vi "RSZVB Delete All Pulse Train Segments.vi"(8 "error in (no error)":errorcluster {"code" format="%.0x"}, 10 "Channel (1)":i32=1, 11 "VISA session":refnum<visa-resource-name>) -> (0 "error out":errorcluster {"code" format="%.0x"}, 3 "dup VISA session":refnum<visa-resource-name>)   [LabVIEW 2011]
doc: "This VI deletes all pulse train segments..\n\nNote(s):\n\n(1) This VI is available only with option R&S ZVA-K27.\n\nRemote-control command(s):\n[SENSe<Ch>:]PULSe:GENerator<gen_no>:TRAin:DELete:ALL"
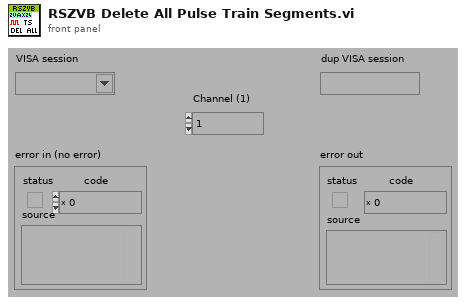
[diagram p1: front panel]
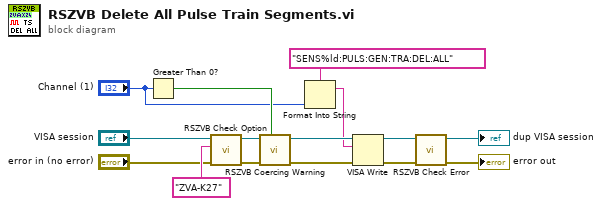
[diagram p0: block diagram]
diagram:
  n1 = Greater Than 0?(x="Channel (1)") -> (x > 0?=w4:bool)
  n2 = call "RSZVB Check Option.vi"("error in (no error)"="error in (no error)", "Options"="ZVA-K27", "VISA session"="VISA session") -> ("error out"=w9:errorcluster, "dup VISA session"=w8:refnum<visa-resource-name>)  [unwired: 7 in]
  n3 = call "RSZVB Coercing Warning.vi"("In Range?"=w4, "error in (no error)"=w9, "VISA session"=w8) -> ("error out"=w14:errorcluster, "dup VISA session"=w15:refnum<visa-resource-name>)  [unwired: 7 in]
  n4 = Format Into String(format string="SENS%ld:PULS:GEN:TRA:DEL:ALL", "Channel (1)") -> (resulting string=w11:string)  [unwired: 2 in, 1 out]
  n5 = VISA Write(VISA resource name=w15, write buffer=w11, error in (no error)=w14) -> (VISA resource name out=w12:refnum<visa-resource-name>, error out=w13:errorcluster)  [unwired: 1 out]
  n6 = call "RSZVB Check Error.vi"("error in (no error)"=w13, "VISA session"=w12) -> ("error out"=→"error out":errorcluster, "dup VISA session"=→"dup VISA session":refnum<visa-resource-name>)  [unwired: 8 in]
